vi "uMsg Defer Reply.vi"(8 "error in (no error)":errorcluster, 11 "uMsg in":refnum<class "uMsg.lvclass">) -> (0 "error out":errorcluster, 3 "uMsg out":refnum<class "uMsg.lvclass">)   [LabVIEW 2021, in "uFramework.lvlib" / "uMsg.lvclass"]
doc: "Set flag to abstain from replying to sender if the \"Send reply\" message is called.\nAny \"send reply\" calls will be ignored."
uses:
  uMsg.lvclass
  uMsg.lvclass/uMsg.ctl
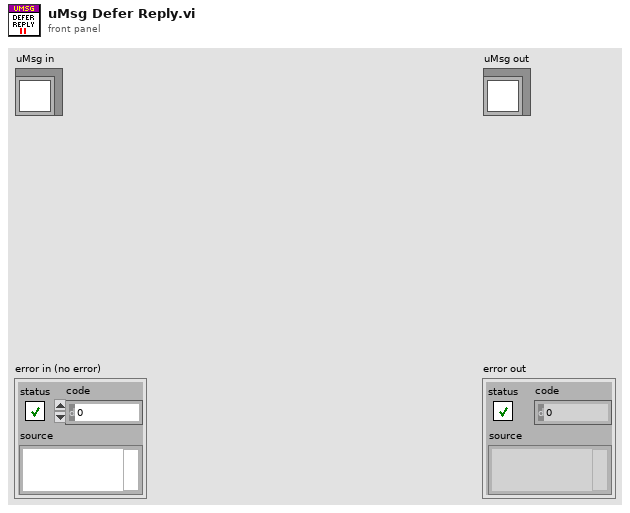
[diagram p1: front panel]
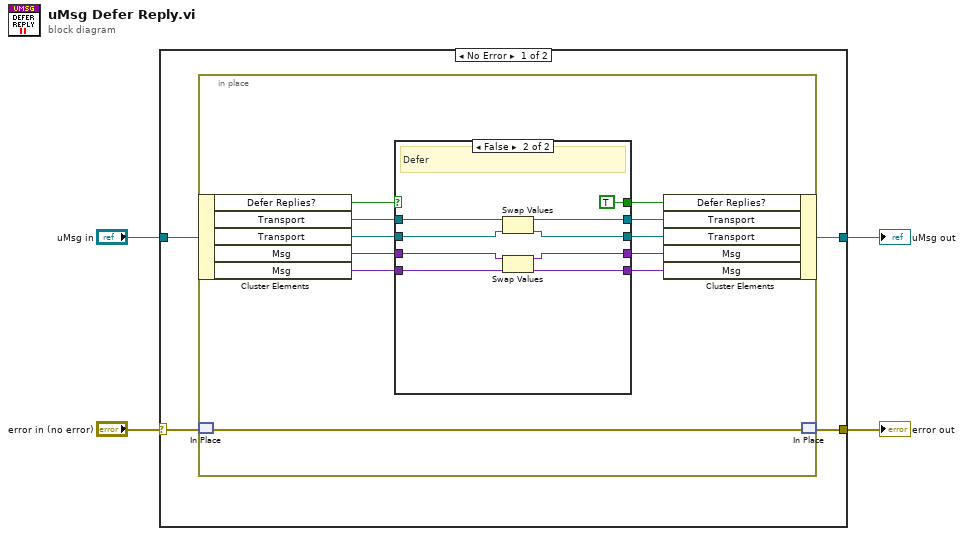
[diagram p0: block diagram]
diagram:
  n1 = case shown="No Error" "error in (no error)" {
    selector: "error in (no error)" -> [w8 w34]
    tunnel: [w7 w34] -> w2
    tunnel: [w5 w35] -> w1
    tunnel: "uMsg in" -> [w6 w35]
    frame No Error {
      n2 = in-place {
        n3 = in-place-cluster #1(w6) -> ("Defer Replies?"=w18:bool, "Transport"=w13:refnum<class "uTransport.lvclass">, "Transport"=w14:refnum<class "uTransport.lvclass">, "Msg"=w15:variant, "Msg"=w16:variant)
        n4 = in-place-match #2(w8) -> (w19:errorcluster)
        n5 = case shown="False" w18 {
          selector: w18 -> [w24 _]
          tunnel: [w24 TRUE] -> w17
          tunnel: w16 -> [w20 w28]
          tunnel: w15 -> [w21 w25]
          tunnel: w14 -> [w22 w31]
          tunnel: w13 -> [w23 w32]
          tunnel: [w23 w30] -> w12
          tunnel: [w22 w29] -> w11
          tunnel: [w21 w26] -> w10
          tunnel: [w20 w27] -> w9
          frame True {
            # "Already Deferred"
          }
          frame False {
            # "Defer"
            n6 = Swap Values(12:w32, 14:w31) -> (1:w30:refnum<class "uTransport.lvclass">, 3:w29:refnum<class "uTransport.lvclass">)  [unwired: 1 in]
            n7 = Swap Values(12:w25, 14:w28) -> (1:w26:variant, 3:w27:variant)  [unwired: 1 in]
          }
        }
        n8 = in-place-cluster #1("Defer Replies?"=w17, "Transport"=w12, "Transport"=w11, "Msg"=w10, "Msg"=w9) -> (w5:refnum<class "uMsg.lvclass">)
        n9 = in-place-match #2(w19) -> (w7:errorcluster)
      }
    }
    frame Error {
    }
  }
  "error out" <- w2
  "uMsg out" <- w1
